vi "add attributs.vi"(8 "error in (no error)":errorcluster caption="entrée d'erreur (pas d'erreur)", 10 "Read/Write":bool, 11 "UI SA en entrée":refnum<class "UI SmarAct.lvclass">) -> (0 "error out":errorcluster caption="sortie d'erreur", 3 "UI SA en sortie":refnum<class "UI SmarAct.lvclass">)   [LabVIEW 2024, in "UI SmarAct.lvclass"]
uses:
  UI SmarAct.lvclass
  Response Cases_Mod.ctl
  UI SmarAct.lvclass/UI SmarAct.ctl
  8f868f25-61c3-40cc-a4bf-92a166941728.vi
  8f868f25-61c3-40cc-a4bf-92a166941728.vi/659df739-fa42-474c-bf03-f9ba45f35773.vi
  <userlib>/LV-TOML/lib/Write TOML File (LV).vi
  <userlib>/LV-TOML/lib/Parse TOML String.vi
  <userlib>/LV-TOML/lib/TOML to LabVIEW.vi
  <userlib>/LV-TOML/lib/LV-TOML.lvlib
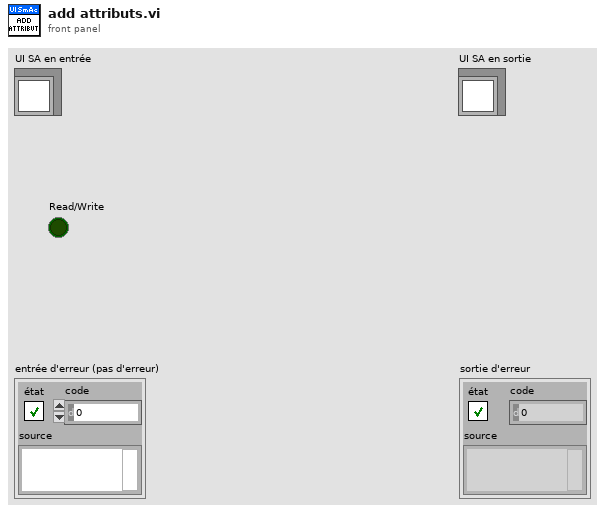
[diagram p1: front panel]
types:
  T1 = typedef "UI SmarAct.lvclass/Response Cases_Mod.ctl" = cluster{"Placeholder - Can be deleted":string, "Channel":u32, "chemin fichier init":path, "max freq (50 ... 18 500)":u32, "speed (0 ... 100 000 000)":u32, "Abs/Rel":bool, "Tps Int(ms)":u32, "Modèle Platine":string, "Début (um)":i32, "fin (um)":i32, "Inc:(um)":string, "Platine Switch":bool, "Port COM":string, "Calib?":bool, "Inc Scan:(um)":string}
  T2 = typedef "UI SmarAct.lvclass/Response Cases.ctl" = cluster{"Placeholder - Can be deleted":string, "Channel":u32, "chemin fichier init":path, "max freq (50 ... 18 500)":u32, "speed (0 ... 100 000 000)":u32, "Abs/Rel":bool, "Tps Int(ms)":u32, "Modèle Platine":string, "Début (um)":i32, "fin (um)":i32, "Inc:(um)":dbl, "Platine Switch":bool, "Port COM":refnum<visa-resource-name>, "Calib?":bool, "Inc Scan:(um)":dbl}
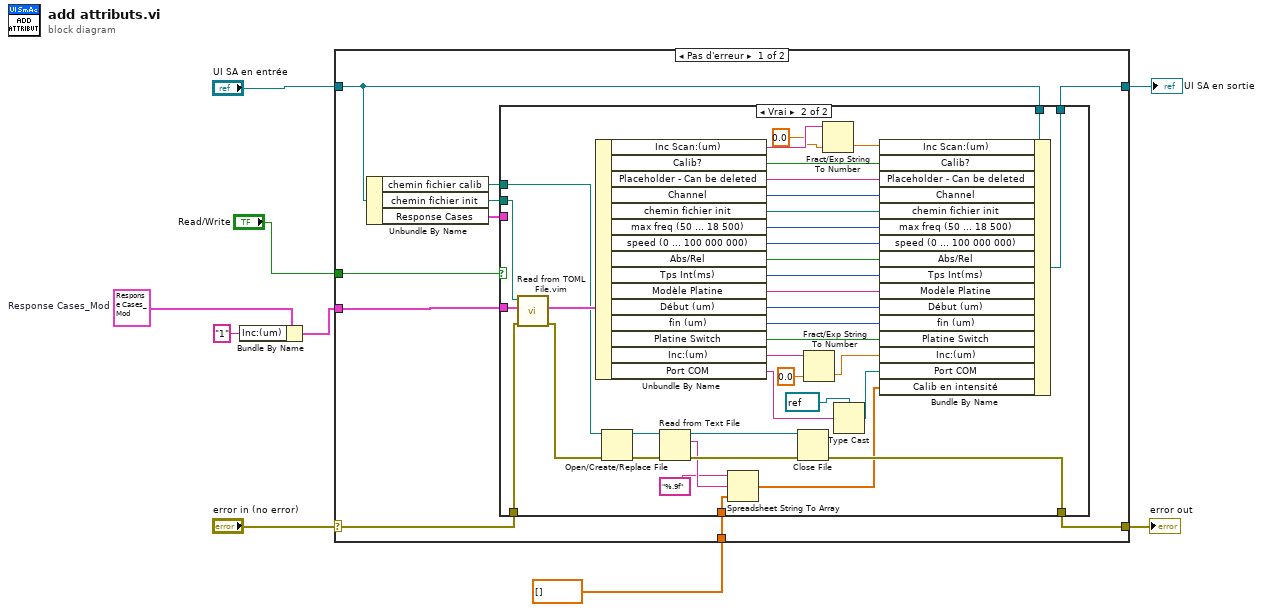
[diagram p0: block diagram]
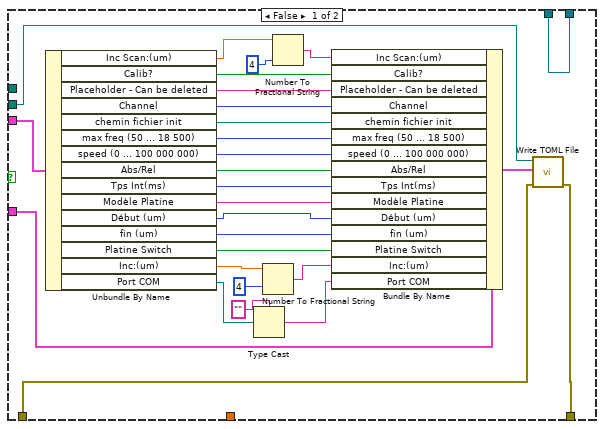
[diagram p2: hidden frame]
diagram:
  w4 = T1 {"Placeholder - Can be deleted"="", "Channel"=0, "chemin fichier init"=path "", "max freq (50 ... 18 500)"=200, "speed (0 ... 100 000 000)"=1000000, "Abs/Rel"=FALSE, "Tps Int(ms)"=0, "Modèle Platine"="", "Début (um)"=0, "fin (um)"=0, "Inc:(um)"="", "Platine Switch"=FALSE, "Port COM"="", "Calib?"=FALSE, "Inc Scan:(um)"=""}  # Response Cases_Mod
  n1 = Bundle By Name(cluster=w4, "Inc:(um)"="1") -> (w3:T1)
  n2 = case shown="Pas d'erreur" "error in (no error)" {
    selector: "error in (no error)" -> [w15 w87]
    tunnel: [w14 w87] -> w8
    tunnel: [w16 w86] -> w6
    tunnel: "UI SA en entrée" -> [w17 w86]
    tunnel: w3 -> [w19 _]
    tunnel: "Read/Write" -> [w13 _]
    tunnel: dbl[] [] -> [w10 _]
    frame No Error {
      n3 = Unbundle By Name(w17) -> ("chemin fichier calib"=w11:path, "chemin fichier init"=w18:path, "Response Cases"=w12:T2)
      n4 = case shown="Vrai" w13 {
        tunnel: w19 -> [w45 w84]
        tunnel: w18 -> [w44 w83]
        tunnel: w17 -> [w46 w82]
        tunnel: [w46 w81] -> w16
        tunnel: w15 -> [w29 w77]
        tunnel: [w30 w58] -> w14
        tunnel: w12 -> [w47 _]
        tunnel: w11 -> [_ w55]
        tunnel: w10 -> [_ w53]
        frame False {
          n5 = Unbundle By Name(w47) -> ("Inc Scan:(um)"=w20:dbl, "Calib?"=w23:bool, "Placeholder - Can be deleted"=w43:string, "Channel"=w40:u32, "chemin fichier init"=w39:path, "max freq (50 ... 18 500)"=w38:u32, "speed (0 ... 100 000 000)"=w37:u32, "Abs/Rel"=w36:bool, "Tps Int(ms)"=w35:u32, "Modèle Platine"=w34:string, "Début (um)"=w33:i32, "fin (um)"=w32:i32, "Platine Switch"=w28:bool, "Inc:(um)"=w42:dbl, "Port COM"=w25:refnum<visa-resource-name>)
          n6 = Type Cast(type="", x=w25) -> (*(type *) &x=w24:string)
          n7 = Number To Fractional String(number=w42, precision (6)=i16 4 ("précision (6)")) -> (F-format string=w41:string)  [unwired: 2 in]
          n8 = Number To Fractional String(number=w20, precision (6)=i16 4 ("précision (6)")) -> (F-format string=w22:string)  [unwired: 2 in]
          n9 = Bundle By Name(cluster=w45, "Inc Scan:(um)"=w22, "Calib?"=w23, "Placeholder - Can be deleted"=w43, "Channel"=w40, "chemin fichier init"=w39, "max freq (50 ... 18 500)"=w38, "speed (0 ... 100 000 000)"=w37, "Abs/Rel"=w36, "Tps Int(ms)"=w35, "Modèle Platine"=w34, "Début (um)"=w33, "fin (um)"=w32, "Platine Switch"=w28, "Inc:(um)"=w41, "Port COM"=w24) -> (w31:T1)
          n10 = call-poly <userlib>:"Write TOML File.vi"("error in (no error)"=w29, "Value"=w31, "file path (use dialog)"=w44) -> ("error out"=w30:errorcluster)  [unwired: 8 in]
        }
        frame True {
          n11 = call "Read from TOML File.vim"("error in (no error)"=w77, "Default Value"=w84, "file path (use dialog)"=w83) -> ("error out"=w61:errorcluster, "Value"=w85:T1)  [unwired: 6 in, 1 out]
          n12 = Unbundle By Name(w85) -> ("Inc Scan:(um)"=w49:string, "Calib?"=w62:bool, "Placeholder - Can be deleted"=w67:string, "Channel"=w68:u32, "chemin fichier init"=w69:path, "max freq (50 ... 18 500)"=w70:u32, "speed (0 ... 100 000 000)"=w71:u32, "Abs/Rel"=w72:bool, "Tps Int(ms)"=w73:u32, "Modèle Platine"=w74:string, "Début (um)"=w75:i32, "fin (um)"=w76:i32, "Platine Switch"=w66:bool, "Inc:(um)"=w80:string, "Port COM"=w64:string)
          n13 = Open/Create/Replace File(file path (use dialog)=w55, error in=w61) -> (refnum out=w57:refnum<file>, error out=w60:errorcluster)  [unwired: 4 in, 1 out]
          n14 = Read from Text File(file (use dialog)=w57, error in=w60) -> (refnum out=w56:refnum<file>, text=w54:string, error out=w59:errorcluster)  [unwired: 2 in, 1 out]
          n15 = Spreadsheet String To Array(format string="%.9f" ("chaîne de format"), spreadsheet string=w54, array type (2D Dbl)=w53) -> (array=w52:dbl[])  [unwired: 1 in]
          n16 = Close File(refnum=w56, error in=w59) -> (error out=w58:errorcluster)  [unwired: 1 out]
          n17 = Fract/Exp String To Number(string=w80, default (0 dbl)=0.0 ("valeur par défaut (0 DBL)")) -> (number=w79:dbl)  [unwired: 2 in, 1 out]
          n18 = Fract/Exp String To Number(string=w49, default (0 dbl)=0.0 ("valeur par défaut (0 DBL)")) -> (number=w50:dbl)  [unwired: 2 in, 1 out]
          n19 = Type Cast(type=refnum<visa-resource-name> refnum ("Response Cases.Port COM"), x=w64) -> (*(type *) &x=w63:refnum<visa-resource-name>)
          n20 = Bundle By Name(cluster=w82, "Inc Scan:(um)"=w50, "Calib?"=w62, "Placeholder - Can be deleted"=w67, "Channel"=w68, "chemin fichier init"=w69, "max freq (50 ... 18 500)"=w70, "speed (0 ... 100 000 000)"=w71, "Abs/Rel"=w72, "Tps Int(ms)"=w73, "Modèle Platine"=w74, "Début (um)"=w75, "fin (um)"=w76, "Platine Switch"=w66, "Inc:(um)"=w79, "Port COM"=w63, "Calib en intensité"=w52) -> (w81:refnum<class "UI SmarAct.lvclass">)
        }
      }
    }
    frame Error {
    }
  }
  "error out" <- w8
  "UI SA en sortie" <- w6
